vi "NI VeriStand - Reset Custom Device Dependencies.vi"(8 "error in (no error)":errorcluster, 11 "Device Ref in":T1 format="%.0x") -> (0 "error out":errorcluster, 3 "Device Ref out":T1 format="%.0x")   [LabVIEW 2020, in "Custom Device API.lvlib"]
doc: "Removes all dependencies from a custom device. Dependencies are any files, such as DLLs or VIs, that the custom device requires and that you want to deploy to the target along with the custom device."
uses:
  <vilib>/NI VeriStand/Custom Device API/Custom Device API.lvlib
  <vilib>/NI VeriStand/Custom Device API/Custom Device Item Ref.ctl
  555bada7-d9b6-4f59-abe8-bfefc96fcee7.vi
  <vilib>/NI VeriStand/Custom Device API/Custom Device Offline Path.vi
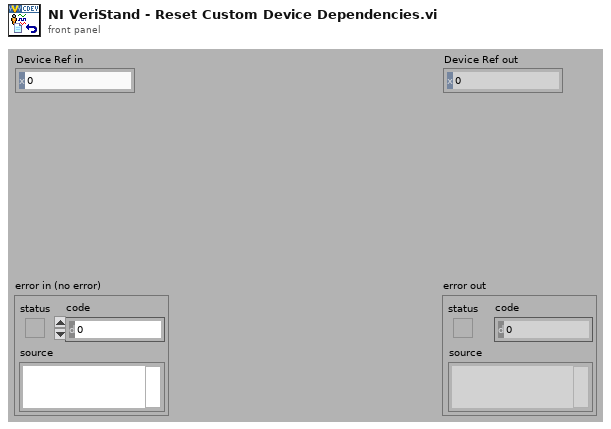
[diagram p1: front panel]
types:
  T1 = typedef "Custom Device API.lvlib/Custom Device Item Ref.ctl" = u64
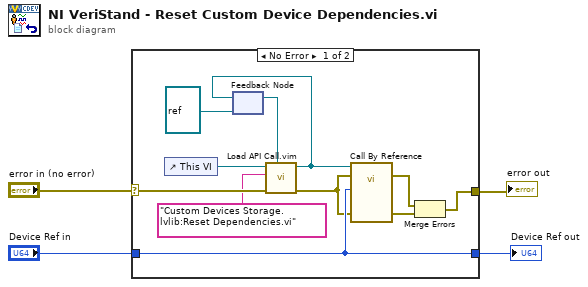
[diagram p0: block diagram]
diagram:
  n1 = case shown="No Error" "error in (no error)" {
    selector: "error in (no error)" -> [w10 w17]
    tunnel: [w14 w17] -> w4
    tunnel: [w13 w16] -> w3
    tunnel: "Device Ref in" -> [w13 w16]
    frame No Error {
      n2 = control-ref of="This VI"() -> (w11:refnum<vi>)
      n3 = feedback #1(refnum<vi> refnum ("type specifier VI Refnum (for type only)")) -> (w12:refnum<vi>)
      n4 = call "Load API Call.vim"("VI reference in"=w12, "error in (no error)"=w10, "VI qualified name"="Custom Devices Storage.lvlib:Reset Dependencies.vi", "Caller VI ref"=w11) -> ("error out"=w9:errorcluster, "VI reference"=w8:refnum<vi>)  [unwired: 6 in]
      n5 = feedback-in #1(w8) -> ()
      n6 = call-by-ref "?"(reference=w8, error in=w9, 8:"error in (no error)"=w9, "Device Ref in"=w13) -> (error out=w5:errorcluster, 0:"error out"=w15:errorcluster)  [unwired: 8 in, 2 out]
      n7 = Merge Errors(w5, w15) -> (w14:errorcluster)
    }
    frame Error {
    }
  }
  "Device Ref out" <- w3
  "error out" <- w4
